vi "XL320_Query Movement.vi"(8 "error in (no error)":errorcluster, 10 "Motor ID (0)":u8, 11 "VISA resource name":refnum<visa-resource-name>) -> (0 "error out":errorcluster, 2 "Motor Moving":bool, 3 "VISA resource name out":refnum<visa-resource-name>)   [LabVIEW 2017, in "Dynamixel XL320.lvlib"]
doc: "Checks to see if the motor is attempting to reach its goal position."
uses:
  <instrlib>/Dynamixel XL320 (Drivers instrument)/Dynamixel XL320.lvlib
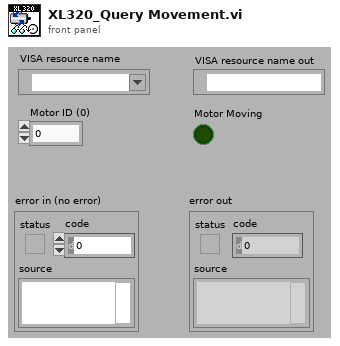
[diagram p1: front panel]
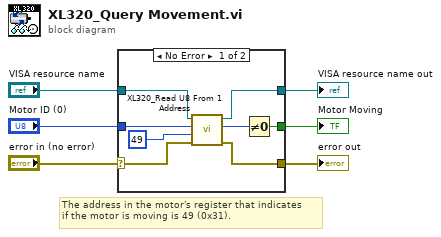
[diagram p0: block diagram]
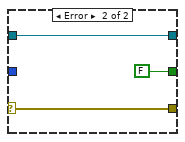
[diagram p2: hidden frame]
diagram:
  # "The address in the motor's register that indicates \nif the motor is moving is 49 (0x31)."
  n1 = case shown="No Error" "error in (no error)" {
    selector: "error in (no error)" -> [w10 w16]
    tunnel: [w14 FALSE] -> w6
    tunnel: "VISA resource name" -> [w13 w17]
    tunnel: [w9 w17] -> w4
    tunnel: [w7 w16] -> w3
    tunnel: "Motor ID (0)" -> [w12 _]
    frame No Error {
      n2 = call <instrlib>:"XL320_Read U8 From 1 Address.vi"("Error in (no error)"=w10, "Address number (0)"=u16 49 ("Address # DEC"), "Motor ID (0)"=w12, "VISA resource name"=w13) -> ("error out"=w7:errorcluster, "Data"=w8:u8, "VISA resource name out"=w9:refnum<visa-resource-name>)  [unwired: 5 in]
      n3 = Not Equal To 0?(x=w8) -> (x != 0?=w14:bool)
    }
    frame Error {
    }
  }
  "VISA resource name out" <- w4
  "error out" <- w3
  "Motor Moving" <- w6
